vi "Convert to TDM or TDMS.vi"(0 "source file path":path, 1 "DataPlugin name":string, 5 "target file path":path, 7 "target file operation (3:create)":T2=enum."create", 9 "target file format (TDMS)":T1=enum."TDMS", 11 "error in (no error)":errorcluster, 12 "data chunk size (1E+7)":i64=10000000 format="%.0e") -> (3 "DataPlugin name out":string, 4 "source file path out":path, 6 "target file path out":path, 15 "error out":errorcluster)   [LabVIEW 2017]
doc: "Converts the specified file to the .tdm or .tdms file format."
uses:
  <vilib>/Platform/storage/lvStorage.llb/_openFunction.ctl
  <vilib>/Platform/storage/utility/usiTDMTDMS.ctl
  <vilib>/Platform/storage/Storage.llb/Get Property (Storage Refnums).vi
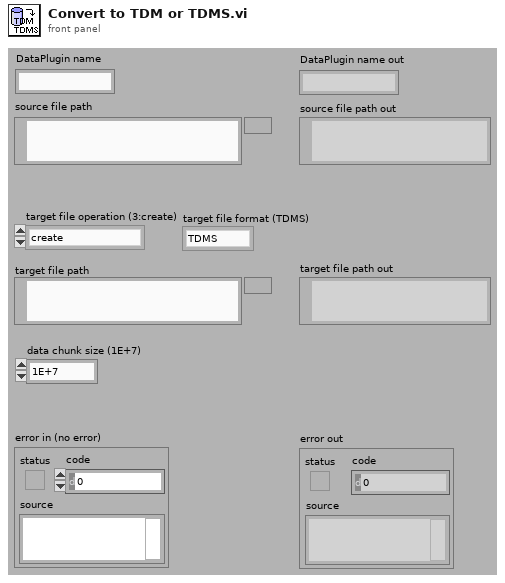
[diagram p1: front panel]
types:
  T1 = typedef "usiTDMTDMS.ctl" = enum16{"TDM", "TDMS"}
  T2 = typedef "_openFunction.ctl" = enum16{"open", "open or create", "create or replace", "create", "open (read only)"}
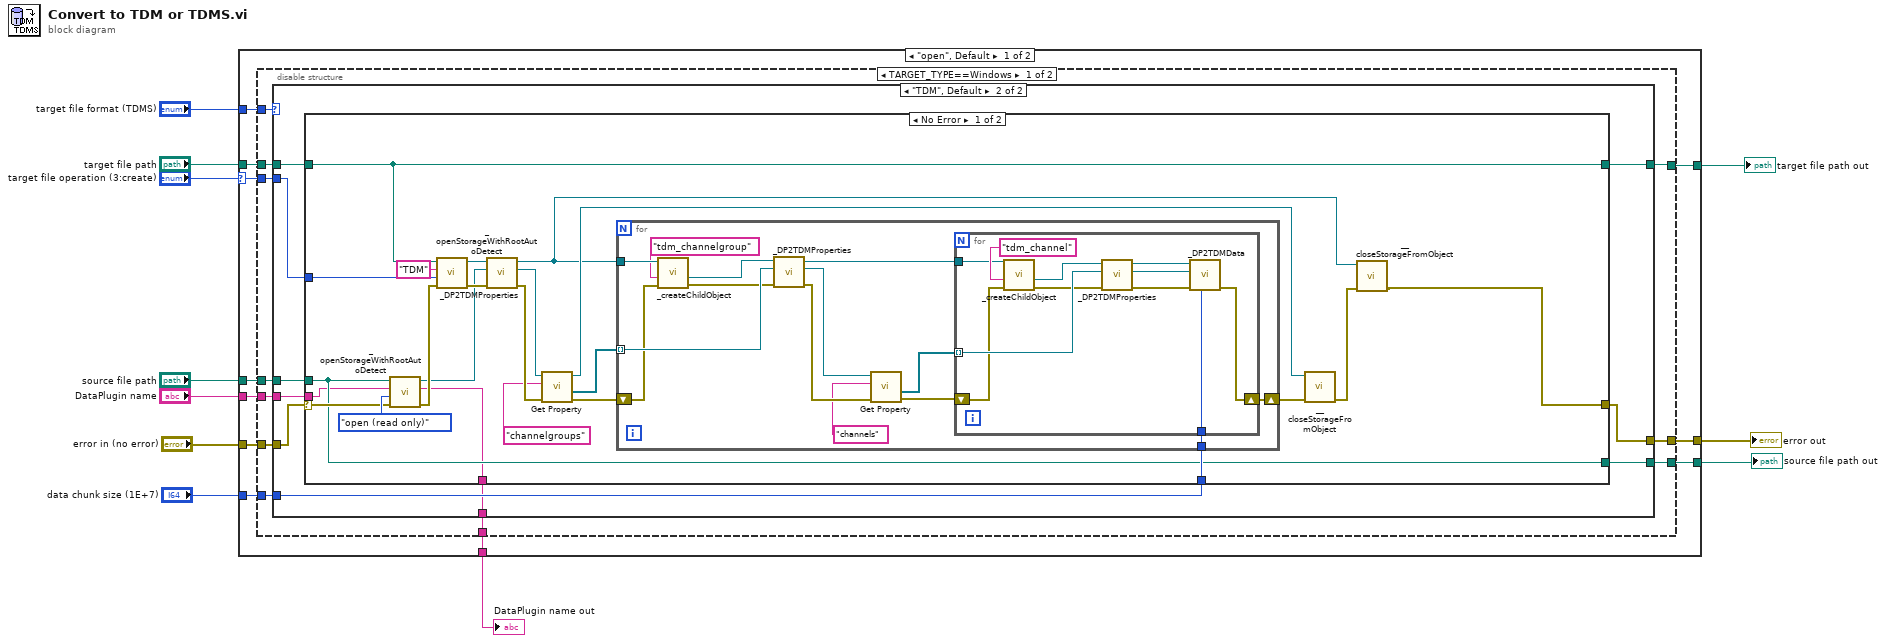
[diagram p0: block diagram]
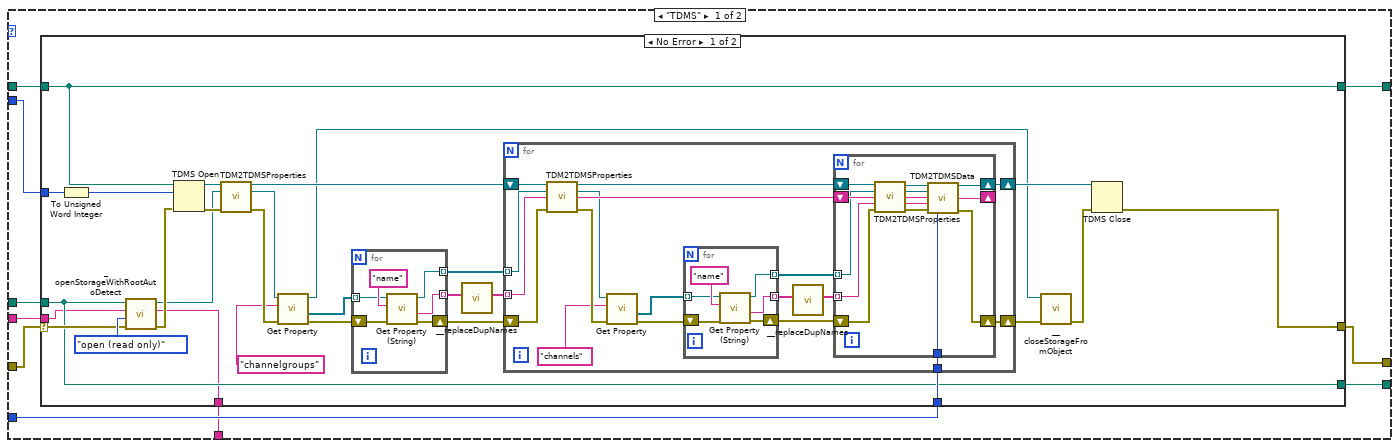
[diagram p2: hidden frame]
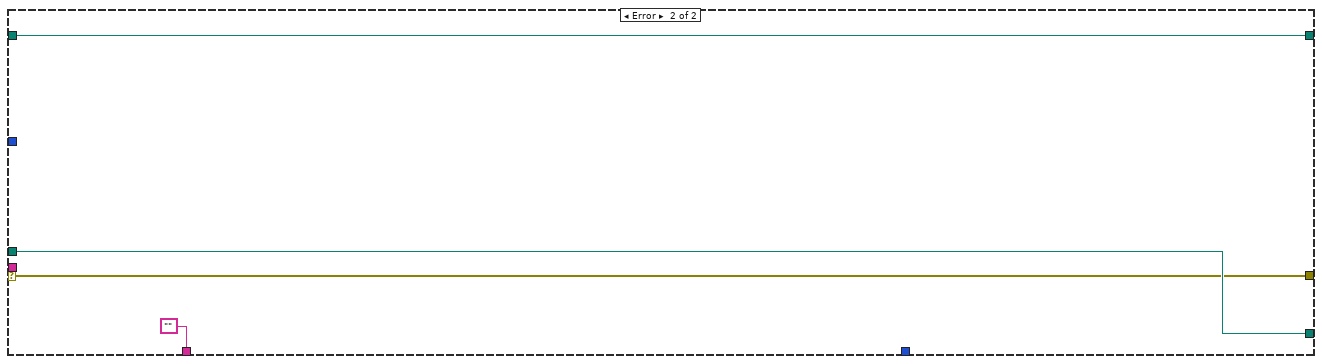
[diagram p3: hidden frame]
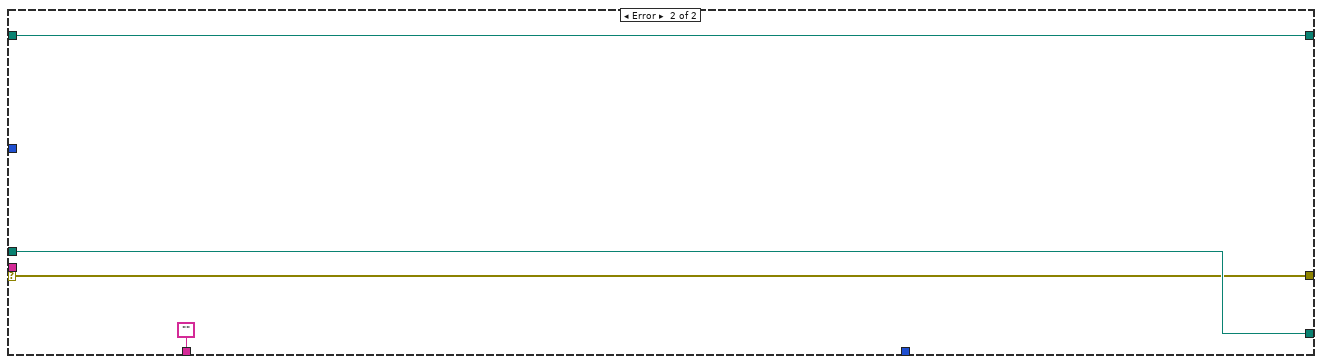
[diagram p4: hidden frame]
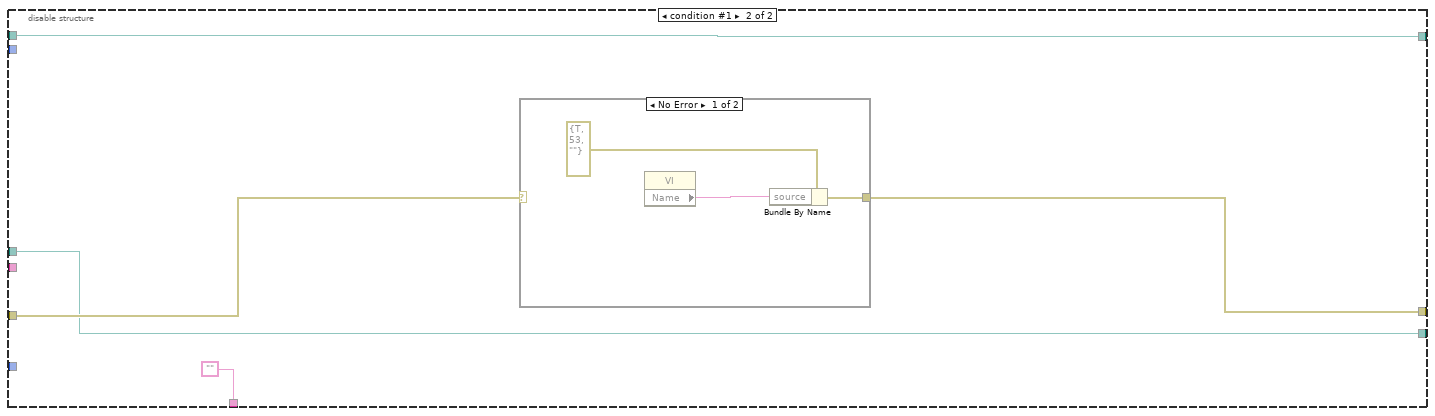
[diagram p5: hidden frame]
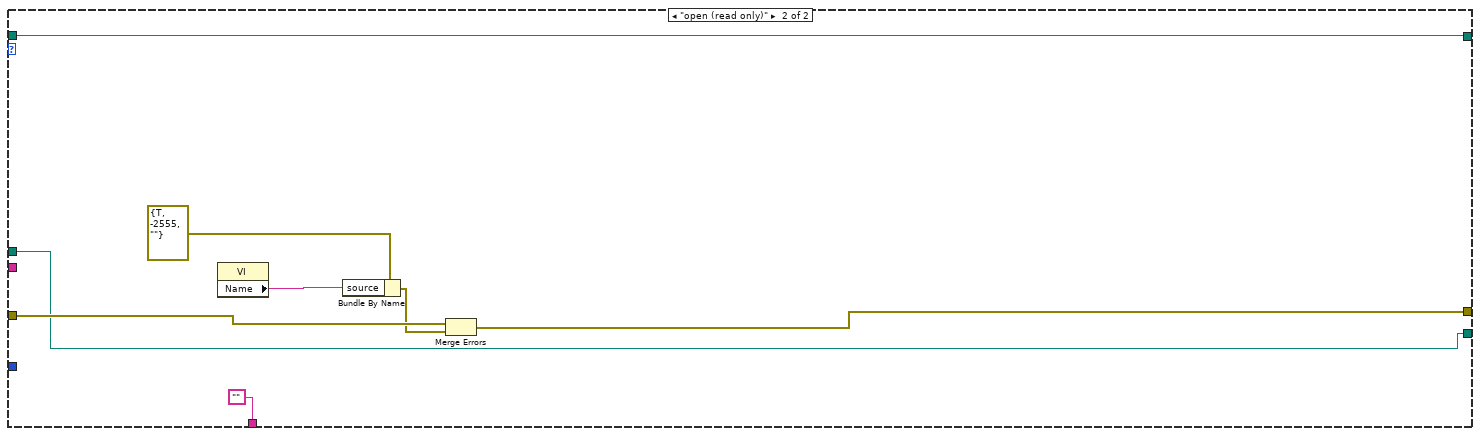
[diagram p7: hidden frame]
diagram:
  n1 = case shown="\"open\", Default" "target file operation (3:create)" {
    selector: "target file operation (3:create)" -> [w19 _]
    tunnel: "target file format (TDMS)" -> [w22 _]
    tunnel: "error in (no error)" -> [w20 w198]
    tunnel: [w15 w197] -> w4
    tunnel: "target file path" -> [w21 w193]
    tunnel: "DataPlugin name" -> [w18 _]
    tunnel: "source file path" -> [w17 w192]
    tunnel: "data chunk size (1E+7)" -> [w16 _]
    tunnel: [w14 w193] -> w3
    tunnel: [w13 w192] -> w2
    tunnel: [w12 "" ("Storage Format out")] -> w1
    frame "open", Default {
      n2 = disable-structure shown="TARGET_TYPE==Windows" {
        disable-tunnel: w22 -> [w33 _]
        disable-tunnel: w21 -> [w32 w184]
        disable-tunnel: w20 -> [w31 w186]
        disable-tunnel: w19 -> [w30 _]
        disable-tunnel: w18 -> [w29 _]
        disable-tunnel: w17 -> [w28 w183]
        disable-tunnel: w16 -> [w27 _]
        disable-tunnel: [w26 w185] -> w15
        disable-tunnel: [w24 w184] -> w14
        disable-tunnel: [w25 w183] -> w13
        disable-tunnel: [w23 "" ("Storage Format out")] -> w12
        frame condition #0 (active) {
          n3 = case shown="\"TDM\", Default" w33 {
            tunnel: w32 -> [w42 w128]
            tunnel: w31 -> [w43 w129]
            tunnel: w30 -> [w41 w127]
            tunnel: w29 -> [w39 w125]
            tunnel: w28 -> [w40 w126]
            tunnel: w27 -> [w38 w124]
            tunnel: [w37 w123] -> w26
            tunnel: [w36 w122] -> w25
            tunnel: [w35 w121] -> w24
            tunnel: [w34 w120] -> w23
            frame "TDMS" {
              n4 = case shown="No Error" w43 {
                selector: w43 -> [w63 w117]
                tunnel: w41 -> [w69 _]
                tunnel: [w44 w117] -> w37
                tunnel: w40 -> [w60 w118]
                tunnel: w42 -> [w59 w119]
                tunnel: [w59 w119] -> w35
                tunnel: [w60 w118] -> w36
                tunnel: w38 -> [w61 _]
                tunnel: w39 -> [w46 _]
                tunnel: [w45 "" ("Storage Format out")] -> w34
                frame No Error {
                  n5 = To Unsigned Word Integer(number=w69) -> (unsigned 16bit integer=w47:u16)
                  n6 = call <vilib>:"_openStorageWithRootAutoDetect.vi"("error in (no error)"=w63, "Overwrite Options"=_openFunction."open (read only)", "Storage Format"=w46, "Storage Location"=w60) -> ("error out"=w62:errorcluster, "Storage Format out"=w45:string, "Data Object"=w54:refnum<k20>)  [unwired: 5 in]
                  n7 = TDMS Open(8:w62, 10:w47, 11:w59) -> (0:w71:errorcluster, 3:w68:refnum<k34>)  [unwired: 4 in]
                  n8 = call <vilib>:"TDM2TDMSProperties.vi"("tdms file in"=w68, "Data Object in"=w54, "error in (no error)"=w71) -> ("tdms file out"=w70:refnum<k34>, "Data Object out"=w58:refnum<k20>, "error out"=w57:errorcluster)  [unwired: 8 in, 2 out]
                  n9 = call-poly <vilib>:"Get Property.vi"("error in (no error)"=w57, "Property name"="channelgroups", "storage refnum"=w58) -> ("error out"=w53:errorcluster, "Value"=w52:refnum<k20>[], "storage refnum out"=w56:refnum<k20>)  [unwired: 6 in]
                  n10 = for {
                    shift-right: [w76] -> w50
                    shift-left: w53 -> [w75]
                    tunnel: w52 -> [w74] mode=indexing
                    tunnel: [w73] -> w51 mode=indexing
                    tunnel: [w72] -> w49 mode=indexing
                    n11 = call <vilib>:"Get Property (String).vi"("error in (no error)"=w75, "Property name"="name", "storage refnum"=w74) -> ("error out"=w76:errorcluster, "Value"=w72:string, "storage refnum out"=w73:refnum<k20>)  [unwired: 6 in]
                  }
                  n12 = call <vilib>:"__replaceDupNames.vi"("input names"=w49) -> ("output names"=w48:string[])  [unwired: 10 in]
                  n13 = for {
                    shift-right: [w92] -> w64
                    shift-left: w70 -> [w94]
                    shift-right: [w95] -> w66
                    shift-left: w50 -> [w79]
                    tunnel: w61 -> [w90]
                    tunnel: w51 -> [w78] mode=indexing
                    tunnel: w48 -> [w80] mode=indexing
                    n14 = call <vilib>:"TDM2TDMSProperties.vi"("tdms file in"=w94, "Data Object in"=w78, "group name"=w80, "error in (no error)"=w79) -> ("tdms file out"=w93:refnum<k34>, "Data Object out"=w87:refnum<k20>, "group name out"=w91:string, "error out"=w89:errorcluster)  [unwired: 7 in, 1 out]
                    n15 = call-poly <vilib>:"Get Property.vi"("error in (no error)"=w89, "Property name"="channels", "storage refnum"=w87) -> ("error out"=w86:errorcluster, "Value"=w85:refnum<k20>[])  [unwired: 6 in, 1 out]
                    n16 = for {
                      shift-right: [w99] -> w84
                      shift-left: w86 -> [w100]
                      tunnel: w85 -> [w98] mode=indexing
                      tunnel: [w97] -> w83 mode=indexing
                      tunnel: [w96] -> w81 mode=indexing
                      n17 = call <vilib>:"Get Property (String).vi"("error in (no error)"=w100, "Property name"="name", "storage refnum"=w98) -> ("error out"=w99:errorcluster, "Value"=w97:string, "storage refnum out"=w96:refnum<k20>)  [unwired: 6 in]
                    }
                    n18 = call <vilib>:"__replaceDupNames.vi"("input names"=w83) -> ("output names"=w82:string[])  [unwired: 10 in]
                    n19 = for {
                      shift-right: [w111] -> w92
                      shift-left: w93 -> [w114]
                      shift-right: [w107] -> w95
                      shift-left: w84 -> [w103]
                      tunnel: w90 -> [w106]
                      shift-right: [w105] -> _
                      shift-left: w91 -> [w115]
                      tunnel: w82 -> [w102] mode=indexing
                      tunnel: w81 -> [w104] mode=indexing
                      n20 = call <vilib>:"TDM2TDMSProperties.vi"("tdms file in"=w114, "Data Object in"=w104, "group name"=w115, "channel name"=w102, "error in (no error)"=w103) -> ("tdms file out"=w113:refnum<k34>, "Data Object out"=w112:refnum<k20>, "group name out"=w109:string, "channel name out"=w108:string, "error out"=w110:errorcluster)  [unwired: 6 in]
                      n21 = call <vilib>:"TDM2TDMSData.vi"("tdms file in"=w113, "storage refnum in"=w112, "group name"=w109, "channel name"=w108, "error in (no error)"=w110, "chunk size"=w106) -> ("tdms file out"=w111:refnum<k34>, "group name out"=w105:string, "error out"=w107:errorcluster)  [unwired: 5 in, 2 out]
                    }
                  }
                  n22 = call <vilib>:"__closeStorageFromObject.vi"("error in (no error)"=w66, "storage refnum"=w56) -> ("error out"=w65:errorcluster)  [unwired: 5 in]
                  n23 = TDMS Close(8:w65, 11:w64) -> (0:w44:errorcluster)  [unwired: 1 out]
                }
                frame Error {
                }
              }
            }
            frame "TDM", Default {
              n24 = case shown="No Error" w129 {
                selector: w129 -> [w150 w179]
                tunnel: w127 -> [w144 _]
                tunnel: [w130 w179] -> w123
                tunnel: w126 -> [w148 w180]
                tunnel: w128 -> [w145 w181]
                tunnel: [w145 w181] -> w121
                tunnel: [w148 w180] -> w122
                tunnel: w124 -> [w149 _]
                tunnel: w125 -> [w146 _]
                tunnel: [w133 "" ("Storage Format out")] -> w120
                frame No Error {
                  n25 = call <vilib>:"_openStorageWithRootAutoDetect.vi"("error in (no error)"=w150, "Overwrite Options"=_openFunction."open (read only)", "Storage Format"=w146, "Storage Location"=w148) -> ("error out"=w142:errorcluster, "Storage Format out"=w133:string, "Data Object"=w139:refnum<k20>)  [unwired: 5 in]
                  n26 = call <vilib>:"_openStorageWithRootAutoDetect.vi"("error in (no error)"=w142, "Overwrite Options"=w144, "Storage Format"="TDM", "Storage Location"=w145) -> ("error out"=w141:errorcluster, "Data Object"=w140:refnum<k20>)  [unwired: 5 in, 1 out]
                  n27 = call <vilib>:"_DP2TDMProperties.vi"("error in (no error)"=w141, "DataPlugin Object in"=w139, "TDM Object in"=w140) -> ("error out"=w138:errorcluster, "DataPlugin object out"=w137:refnum<k20>, "TDM Object out"=w131:refnum<k20>)  [unwired: 6 in]
                  n28 = call-poly <vilib>:"Get Property.vi"("error in (no error)"=w138, "Property name"="channelgroups", "storage refnum"=w137) -> ("error out"=w132:errorcluster, "Value"=w135:refnum<k20>[], "storage refnum out"=w147:refnum<k20>)  [unwired: 6 in]
                  n29 = for {
                    shift-right: [w166] -> w151
                    shift-left: w132 -> [w158]
                    tunnel: w149 -> [w165]
                    tunnel: w135 -> [w164] mode=indexing
                    tunnel: w131 -> [w159]
                    n30 = call <vilib>:"_createChildObject.vi"("error in (no error)"=w158, "Object type"="tdm_channelgroup", "storage refnum"=w159) -> ("error out"=w156:errorcluster, "new storage refnum"=w155:refnum<k20>)  [unwired: 2 in, 1 out]
                    n31 = call <vilib>:"_DP2TDMProperties.vi"("error in (no error)"=w156, "DataPlugin Object in"=w164, "TDM Object in"=w155) -> ("error out"=w163:errorcluster, "DataPlugin object out"=w162:refnum<k20>, "TDM Object out"=w153:refnum<k20>)  [unwired: 6 in]
                    n32 = call-poly <vilib>:"Get Property.vi"("error in (no error)"=w163, "Property name"="channels", "storage refnum"=w162) -> ("error out"=w154:errorcluster, "Value"=w160:refnum<k20>[])  [unwired: 6 in, 1 out]
                    n33 = for {
                      shift-right: [w174] -> w166
                      shift-left: w154 -> [w171]
                      tunnel: w165 -> [w176]
                      tunnel: w160 -> [w177] mode=indexing
                      tunnel: w153 -> [w167]
                      n34 = call <vilib>:"_createChildObject.vi"("error in (no error)"=w171, "Object type"="tdm_channel", "storage refnum"=w167) -> ("error out"=w169:errorcluster, "new storage refnum"=w168:refnum<k20>)  [unwired: 2 in, 1 out]
                      n35 = call <vilib>:"_DP2TDMProperties.vi"("error in (no error)"=w169, "DataPlugin Object in"=w177, "TDM Object in"=w168) -> ("error out"=w175:errorcluster, "DataPlugin object out"=w172:refnum<k20>, "TDM Object out"=w173:refnum<k20>)  [unwired: 6 in]
                      n36 = call <vilib>:"_DP2TDMData.vi"("chunk size"=w176, "error in (no error)"=w175, "DataPlugin Object in"=w172, "TDM Object in"=w173) -> ("error out"=w174:errorcluster)  [unwired: 5 in, 2 out]
                    }
                  }
                  n37 = call <vilib>:"__closeStorageFromObject.vi"("error in (no error)"=w151, "storage refnum"=w147) -> ("error out"=w136:errorcluster)  [unwired: 5 in]
                  n38 = call <vilib>:"__closeStorageFromObject.vi"("error in (no error)"=w136, "storage refnum"=w131) -> ("error out"=w130:errorcluster)  [unwired: 5 in]
                }
                frame Error {
                }
              }
            }
          }
        }
        frame condition #1 {
          n39 = case shown="No Error" w186 {
            selector: w186 -> [_ w190]
            tunnel: [w188 w190] -> w185
            frame No Error {
              n40 = property class="VI"() -> ("Name"=w187:string)  [unwired: 2 in, 2 out]
              n41 = Bundle By Name(cluster=errorcluster {"status"=TRUE, "code"=53, "source"=""} ("error IO"), "source"=w187) -> (w188:errorcluster)
            }
            frame Error {
            }
          }
        }
      }
    }
    frame "open (read only)" {
      n42 = property class="VI"() -> ("Name"=w196:string)  [unwired: 2 in, 2 out]
      n43 = Bundle By Name(cluster=errorcluster {"status"=TRUE, "code"=-2555, "source"=""} ("error in 2 (no error)"), "source"=w196) -> (w194:errorcluster)
      n44 = Merge Errors(w198, w194) -> (w197:errorcluster)
    }
  }
  "error out" <- w4
  "source file path out" <- w2
  "target file path out" <- w3
  "DataPlugin name out" <- w1
